vi "Main_08B.vi"() -> ()   [LabVIEW 2024]
uses:
  Map_Antena.ctl
  Cluster_Position.ctl
  <vilib>/Utility/miscctls.llb/LVMapReplaceAction.ctl
panel:
  out "Final Grid":string[][](array[string])
  out "Antena Map":T1
  out "Original Grid":string[][](array[string])
  in  "Use Puzzle":bool
  out "Answer 1115":u32
  in  "Puzzle":string="............s...............1.....................\n......................E......3.....S..............\n.......................3.....S....................\n...e........T.t.......S.1...........I.............\n..................B..................I.....O......\ng.......z........i39......B..I....................\n.......s....S.......3......................i..I...\n....e.............2..........B....................\n.......tC...z.......g......1......................\n.E......s....R....................................\n..G...t..........2................................\n.........K...C.......2............................\n....T..e...........5...C..........................\n...T................................O...o.........\n...............................g..............o...\n.........z...................g......i............o\n...9.E............H...........Y.......O...........\n..........R..H...............7.O..................\n...........H.............v......7........B........\n..9.Q.......................W......1........Y.....\n.........................z.7.................Y....\n.....Q................................v...........\n....K.......E.....R...............2..........o....\n.n............H......v...........................Y\n.G.y..........................Q...................\n......G....A5.....................h...............\n..........D...5.w...9.............................\n......n....5...L..................................\n............................v.....................\n............L...0t..........7.....................\n..n....k............y....................W........\n..k..........0.........................W..........\n...n.......R..L..a........................W.......\n.........................................h........\n..0..L........c...b...............................\n.....................8.y..........................\n.......w.................6.............h.......N..\n..........y..4....................................\n...0....8...k.....Z........r......................\n..............a...8Z.........G......4.............\n........4..b.q.....................K..............\n.q...........kZ.K......b..D.........d.............\n.8.....................D................r.........\n.....w.........a...............d........A.........\n................................d.A.hV............\n................c..........D.....V....r...........\n.......Z......6.....l........................A.d..\n...................l..6..c....b......r...........N\n......a....4........q..l..V..c................N...\nl.....w...........q..6............V..............."
  in  "Example":string="............\n........0...\n.....0......\n.......0....\n....0.......\n......A.....\n............\n............\n........A...\n.........A..\n............\n............"
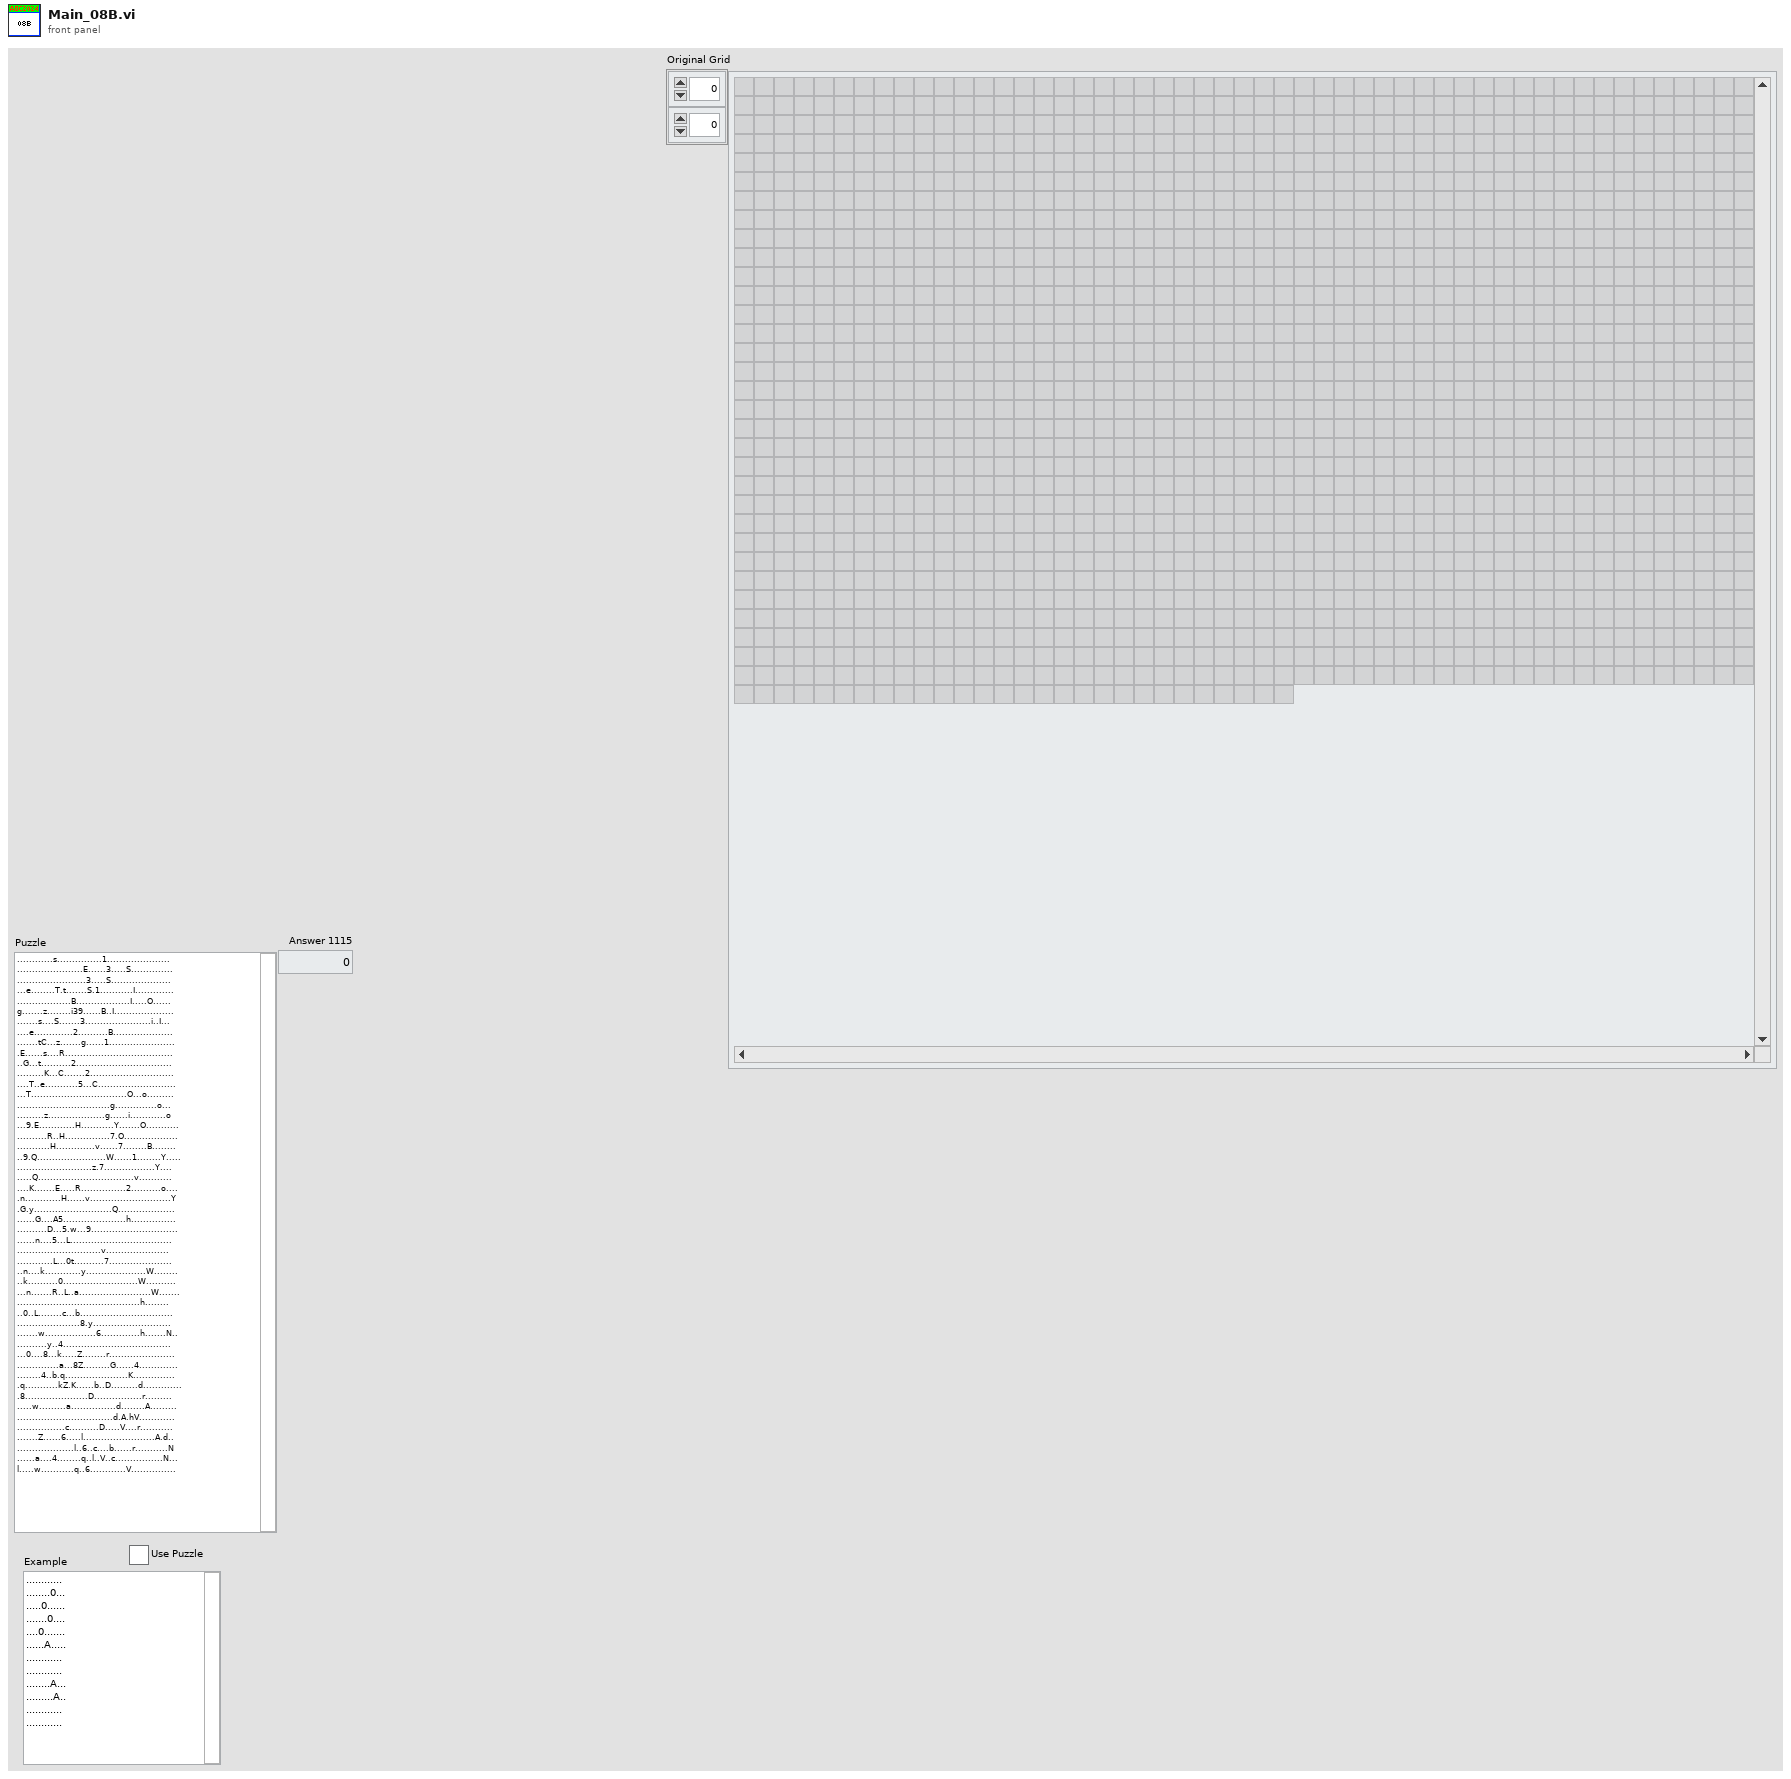
[diagram p1: front panel]
types:
  T1 = typedef "Map_Antena.ctl" = map{string, set{T2}}
  T2 = typedef "Cluster_Position.ctl" = cluster{"R":i32, "C":i32}
  T3 = typedef "LVMapReplaceAction.ctl" = enum32{"Modify Entry only if found", "Add or Modify Entry", "Delete Entry"}
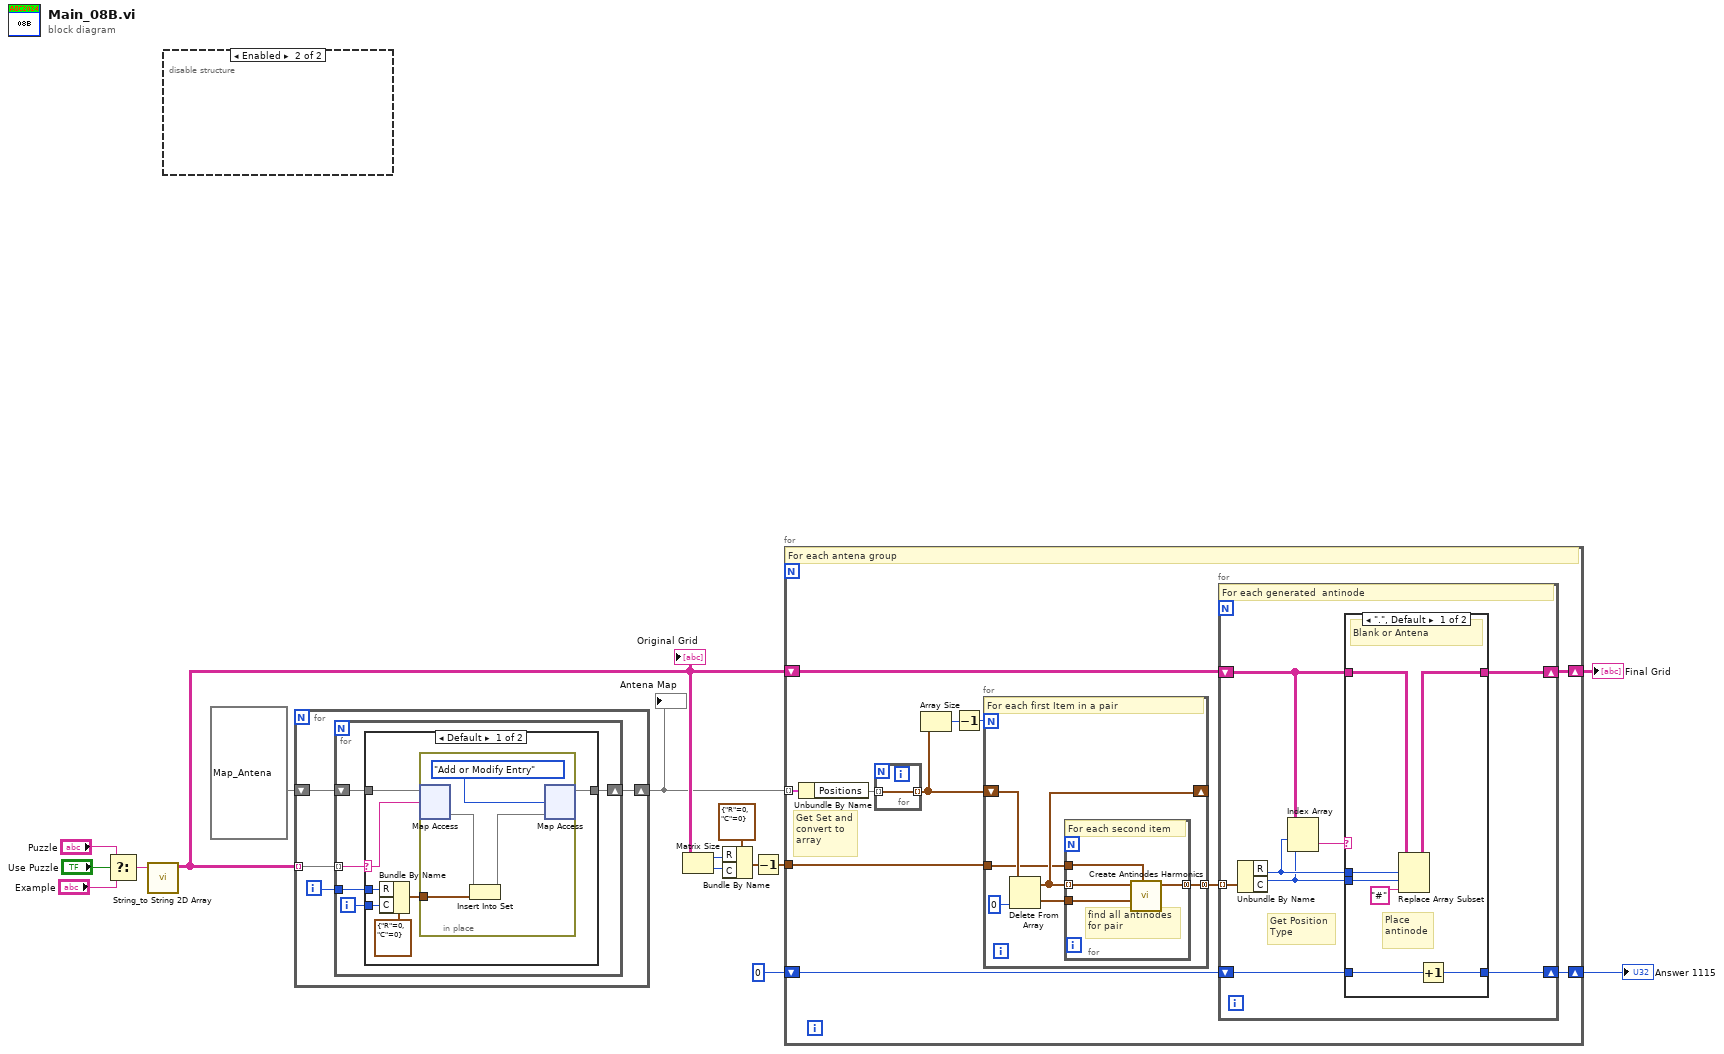
[diagram p0: block diagram]
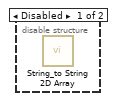
[diagram p3: hidden frame]
diagram:
  n1 = Select(t="Puzzle", s="Use Puzzle", f="Example") -> (s? t:f=w4:string)
  n2 = call "String_to String 2D Array.vi"("Input String"=w4) -> ("2D Array"=w2:string[][])  [unwired: 10 in]
  "Original Grid" <- w2
  n3 = disable-structure shown="Enabled" {
    frame Disabled {
      n4 = call "String_to String 2D Array.vi"() -> ()  [unwired: 11 in, 1 out]
    }
    frame Enabled {
    }
  }
  n5 = for {
    tunnel: w2 -> [w19] mode=indexing
    shift-right: [w17] -> w1
    shift-left: T1 {} ("Antena Map") -> [w18]
    i -> [w16]
    n6 = for {
      tunnel: w19 -> [w24] mode=indexing
      shift-right: [w20] -> w17
      shift-left: w18 -> [w23]
      tunnel: w16 -> [w22]
      i -> [w21]
      n7 = case shown="Default" w24 {
        selector: w24 -> [w30 _]
        tunnel: w23 -> [w31 w36]
        tunnel: w22 -> [w28 _]
        tunnel: w21 -> [w27 _]
        tunnel: [w25 w36] -> w20
        frame Default {
          n8 = Bundle By Name(cluster=T2 {"R"=0, "C"=0} ("Position"), "R"=w28, "C"=w27) -> (w26:T2)
          n9 = in-place {
            in-place-border: w26 -> [w32]
            n10 = in-place-map #1(w31, w30) -> (w34:set{T2})  [unwired: 1 in, 1 out]
            n11 = Insert Into Set(10:w32, 11:w34) -> (3:w33:set{T2})  [unwired: 1 out]
            n12 = in-place-map #1(w33, LVMapReplaceAction."Add or Modify Entry" ("action")) -> (w25:T1)  [unwired: 2 out]
          }
        }
        frame "." {
        }
      }
    }
  }
  "Antena Map" <- w1
  n13 = Matrix Size(0:w2) -> (1:w7:i32, 2:w6:i32)
  n14 = Bundle By Name(cluster=T2 {"R"=0, "C"=0} ("Position"), "R"=w7, "C"=w6) -> (w5:T2)
  n15 = Decrement(x=w5) -> (x-1=w3:T2)
  n16 = for {
    tunnel: w3 -> [w41]
    shift-right: [w43] -> w11
    shift-left: u32 0 -> [w44]
    shift-right: [w42] -> w10
    shift-left: w2 -> [w45]
    tunnel: w1 -> [w39] mode=indexing
    # "Get Set and\nconvert to \narray"
    # "For each antena group"
    n17 = Unbundle By Name(w39) -> ("Positions"=w38:set{T2})
    n18 = for {
      tunnel: w38 -> [w48] mode=indexing
      tunnel: [w48] -> w37 mode=indexing
    }
    n19 = Array Size(array=w37) -> (size(s)=w47:i32)
    n20 = Decrement(x=w47) -> (x-1=w46:i32)
    n21 = for {
      N: w46 -> [_]
      shift-right: [w68] -> _
      shift-left: w37 -> [w71]
      tunnel: [w67] -> w40 mode=concatenating
      tunnel: w41 -> [w66]
      # "For each first Item in a pair"
      n22 = Delete From Array(array=w71, index=0) -> (deleted portion=w69:T2, array with subset deleted=w68:T2[])  [unwired: 1 in]
      n23 = for {
        tunnel: w69 -> [w74]
        tunnel: w68 -> [w75] mode=indexing
        tunnel: [w72] -> w67 mode=concatenating
        tunnel: w66 -> [w73]
        # "find all antinodes\nfor pair"
        # "For each second item"
        n24 = call "Create Antinodes Harmonics.vi"("Max Grid Index"=w73, "Antena 2"=w74, "Antena 1"=w75) -> ("Antinodes"=w72:T2[])  [unwired: 8 in]
      }
    }
    n25 = for {
      shift-right: [w55] -> w42
      shift-left: w45 -> [w56]
      shift-right: [w53] -> w43
      shift-left: w44 -> [w54]
      tunnel: w40 -> [w49] mode=indexing
      # "Get Position\nType"
      # "For each generated  antinode"
      n26 = Unbundle By Name(w49) -> ("R"=w51:i32, "C"=w50:i32)
      n27 = Index Array(array=w56, index (row)=w51, index (col)=w50) -> (element=w52:string)
      n28 = case shown="\".\", Default" w52 {
        tunnel: w56 -> [w63 w65]
        tunnel: w51 -> [w61 _]
        tunnel: w50 -> [w60 _]
        tunnel: [w62 w65] -> w55
        tunnel: w54 -> [w58 w64]
        tunnel: [w57 w64] -> w53
        frame ".", Default {
          # "Place\nantinode"
          # "Blank or Antena"
          n29 = Replace Array Subset(array=w63, new element="#" ("new element/subarray"), index (row)=w61, index (col)=w60) -> (w62:string[][])
          n30 = Increment(x=w58) -> (x+1=w57:u32)
        }
        frame "#" {
          # "Antinode"
        }
      }
    }
  }
  "Answer 1115" <- w11
  "Final Grid" <- w10
